vi "mpps_keithley-2400_python.vi"(0 "start voltage (V)":string, 1 "file name":string, 2 "folder path":string, 5 "nplc":string, 7 "settling delay (s)":string, 9 "total tracking time (s)":string, 11 "error in (no error)":errorcluster, 12 "illumination intensity (suns equiv.)":string, 13 "area (cm^2)":string) -> (15 "error out":errorcluster)   [LabVIEW 2016]
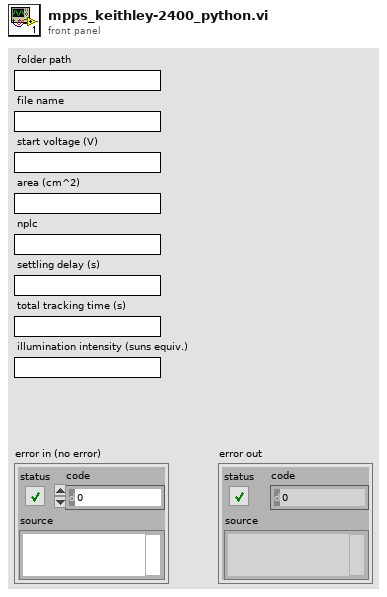
[diagram p1: front panel]
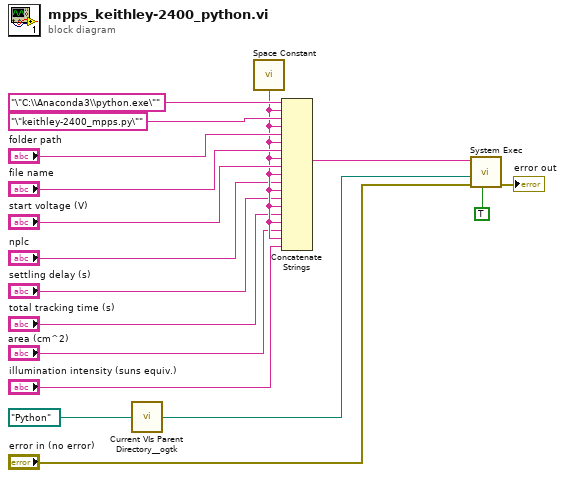
[diagram p0: block diagram]
diagram:
  n1 = call <userlib>:"Current VIs Parent Directory__ogtk.vi"("Relative path (.)"=path "Python") -> ("Parent Directory (+ Relative)"=w7:path)  [unwired: 4 in]
  n2 = call <vilib>:"Space Constant.vi"() -> ("String"=w9:string)
  n3 = Concatenate Strings("\"C:\\Anaconda3\\python.exe\"" ("standard input"), w9, "\"keithley-2400_mpps.py\"" ("standard input"), w9, "folder path", w9, "file name", w9, "start voltage (V)", w9, "nplc", w9, "settling delay (s)", w9, "total tracking time (s)", w9, "area (cm^2)", w9, "illumination intensity (suns equiv.)") -> (w15:string)
  n4 = call <vilib>:"System Exec.vi"("run minimized? (F)"=TRUE, "error in (no error)"="error in (no error)", "working directory"=w7, "command line"=w15) -> ("error out"=→"error out":errorcluster)  [unwired: 4 in, 3 out]
